vi "DoubleSolenoidCommandState.vi"(0 "Device Reference (in)":T2, 5 "Output Mode":T1(ring), 9 "State [True, False]":bool, 11 "Error (in)":errorcluster) -> ()   [LabVIEW 2020]
doc: "Wrapper for commanding the state of a double-acting solenoid. Supports the standard actuator testing interface and only sending commands on change."
uses:
  <vilib>/Rock Robotics/WPI/Solenoid/Deprecated/WPI_SolenoidSetBool.vi
  <vilib>/Rock Robotics/WPI/Solenoid/WPI_SolenoidChannel.ctl
  <vilib>/Rock Robotics/WPI/Solenoid/WPI_SolenoidDevRef.ctl
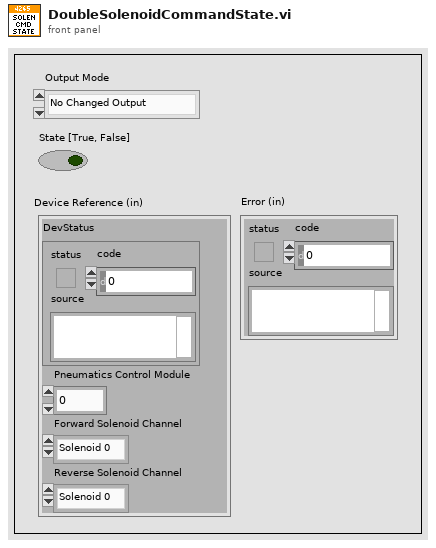
[diagram p1: front panel]
types:
  T1 = enum16{"No Changed Output", "New Normal Output", "New Testing Output"}
  T2 = typedef "WPI_SolenoidDevRef.ctl" = cluster{"DevStatus":errorcluster, "Pneumatics Control Module":u8, "Forward Solenoid Channel":T3, "Reverse Solenoid Channel":T3}
  T3 = typedef "WPI_SolenoidChannel.ctl" = enum8{"Solenoid 0", "Solenoid 1", "Solenoid 2", "Solenoid 3", "Solenoid 4", "Solenoid 5", "Solenoid 6", "Solenoid 7", "Solenoid 8", "Solenoid 9", "Solenoid 10", "Solenoid 11", "Solenoid 12", "Solenoid 13", "Solenoid 14", "Solenoid 15", "Invalid"}
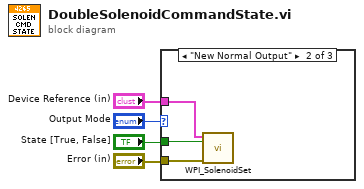
[diagram p0: block diagram]
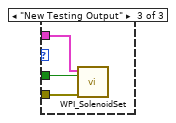
[diagram p3: hidden frame]
diagram:
  n1 = case shown="\"New Normal Output\"" "Output Mode" {
    tunnel: "State [True, False]" -> [_ w6 w9]
    tunnel: "Device Reference (in)" -> [_ w7 w10]
    tunnel: "Error (in)" -> [_ w5 w8]
    frame "No Changed Output", Default {
    }
    frame "New Normal Output" {
      n2 = call-poly <vilib>:"WPI_SolenoidSet.vi"("error in (no error)"=w5, "Value"=w6, "SolenoidDevRef"=w7) -> ()  [unwired: 7 in, 2 out]
    }
    frame "New Testing Output" {
      n3 = call-poly <vilib>:"WPI_SolenoidSet.vi"("error in (no error)"=w8, "Value"=w9, "SolenoidDevRef"=w10) -> ()  [unwired: 7 in, 2 out]
    }
  }
